vi "Write Results File.vi"(5 "Timing Stats":T1, 7 "All Roundtrip Measurments (usec)":string, 8 "error in (no error)":errorcluster, 11 "Filename":string) -> (0 "error out":errorcluster)   [LabVIEW 2021]
uses:
  TYPEDEF - Overall Timing Statistics.ctl
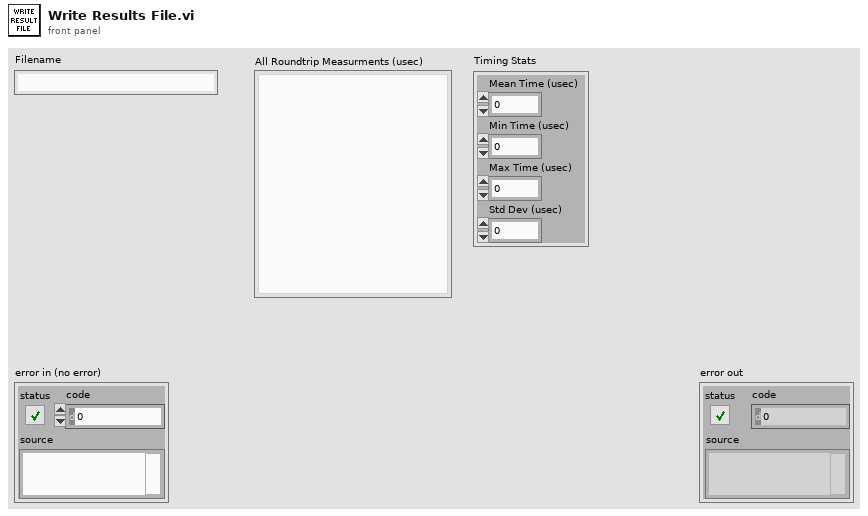
[diagram p1: front panel]
types:
  T1 = typedef "TYPEDEF - Overall Timing Statistics.ctl" = cluster{"Mean Time (usec)":dbl, "Min Time (usec)":dbl, "Max Time (usec)":dbl, "Std Dev (usec)":dbl}
  T2 = enum16{"open", "replace", "create", "open or create", "replace or create", "replace or create with confirmation"}
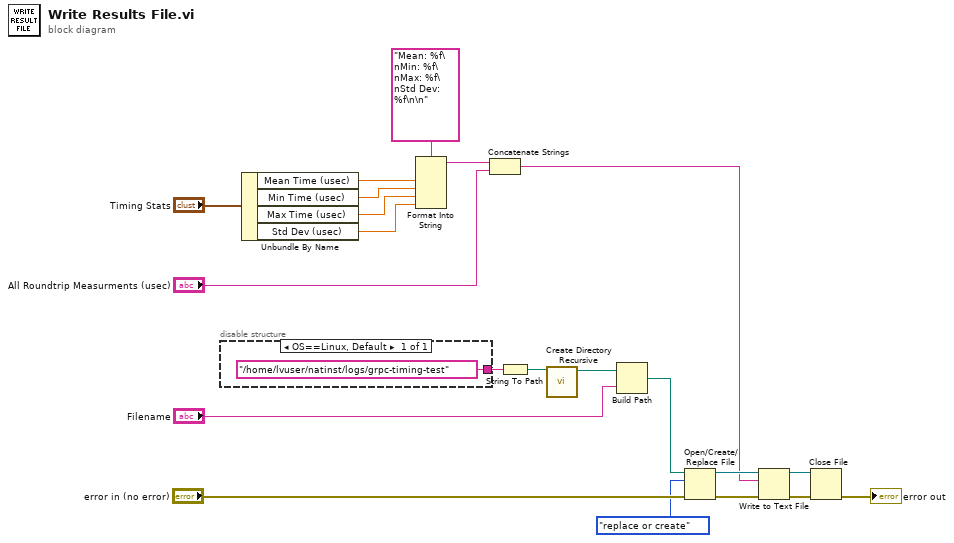
[diagram p0: block diagram]
diagram:
  n1 = disable-structure shown="OS==Linux, Default" {
    disable-tunnel: ["/home/lvuser/natinst/logs/grpc-timing-test"] -> w15
    frame condition #0 (active) {
    }
  }
  n2 = Unbundle By Name("Timing Stats") -> ("Mean Time (usec)"=w9:dbl, "Min Time (usec)"=w8:dbl, "Max Time (usec)"=w7:dbl, "Std Dev (usec)"=w6:dbl)
  n3 = Format Into String(format string="Mean: %f\nMin: %f\nMax: %f\nStd Dev: %f\n\n", w9, w8, w7, w6) -> (resulting string=w4:string)  [unwired: 2 in, 1 out]
  n4 = Concatenate Strings(w4, "All Roundtrip Measurments (usec)") -> (w2:string)
  n5 = String To Path(string=w15) -> (path=w14:path)
  n6 = call <vilib>:"Create Directory Recursive.vi"("directory"=w14) -> ("directory copy"=w13:path)  [unwired: 4 in, 2 out]
  n7 = Build Path(base path=w13, name or relative path="Filename") -> (appended path=w11:path)
  n8 = Open/Create/Replace File(file path (use dialog)=w11, error in="error in (no error)", operation (0:open)=T2."replace or create") -> (refnum out=w21:refnum<file>, error out=w20:errorcluster)  [unwired: 3 in, 1 out]
  n9 = Write to Text File(file (use dialog)=w21, text=w2, error in=w20) -> (refnum out=w19:refnum<file>, error out=w18:errorcluster)  [unwired: 1 in, 1 out]
  n10 = Close File(refnum=w19, error in=w18) -> (error out=→"error out":errorcluster)  [unwired: 1 out]
